vi "LabvolutionSubmoduleCheck_HasSubmodules.vi"(7 "Project Path":path=path "C:/Users/GregPayne/Documents/grp/fibre-geometry/Fibre Geometry.lvproj", 11 "Standard Output":string) -> (3 "Submodules exist":bool)   [LabVIEW 2018]
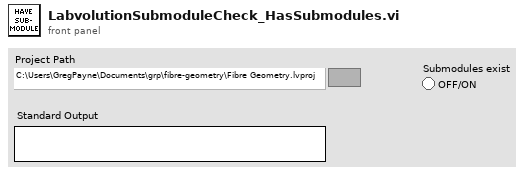
[diagram p1: front panel]
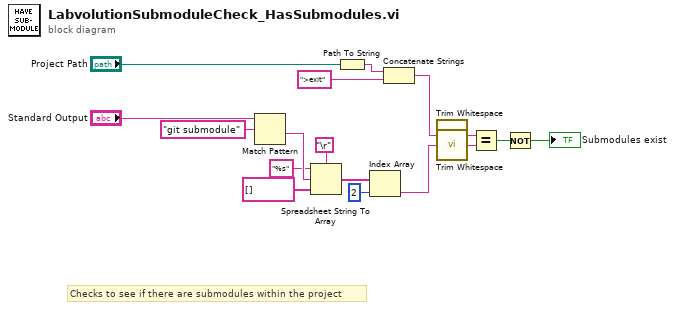
[diagram p0: block diagram]
diagram:
  # "Checks to see if there are submodules within the project"
  n1 = Match Pattern(string="Standard Output", regular expression="git submodule") -> (after substring=w15:string)  [unwired: 1 in, 3 out]
  n2 = Spreadsheet String To Array(delimiter (Tab)="\r", format string="%s", spreadsheet string=w15, array type (2D Dbl)=string[] []) -> (array=w11:string[])
  n3 = Path To String(path="Project Path") -> (string=w9:string)
  n4 = Index Array(array=w11, index=2) -> (element=w6:string)
  n5 = Concatenate Strings(w9, ">exit" ("string")) -> (w7:string)
  n6 = call <vilib>:"Trim Whitespace.vi"("string"=w7) -> ("trimmed string"=w4:string)  [unwired: 1 in]
  n7 = call <vilib>:"Trim Whitespace.vi"("string"=w6) -> ("trimmed string"=w5:string)  [unwired: 1 in]
  n8 = Equal?(x=w4, y=w5) -> (x = y?=w3:bool)
  n9 = Not(x=w3) -> (.not. x?=→"Submodules exist":bool)
